vi "Tx handeset.vi"(0 "CMD On":string, 5 "CMD Off":string, 7 "Set Point":string, 9 "Estado do Botão":bool, 11 "Velocity (arcsec/sec)":dbl(slide) min=0.0 scale=0.0..30.0) -> ()   [LabVIEW 2018]
uses:
  Global Tabs.vi
panel:
  out "Offset":dbl min=0.0 max=360.0
  out "mec position":dbl min=0.0 max=360.0 format="%.2f"
  out "pos (deg)":dbl min=0.0 max=360.0 format="%.2f"
  in  "mec pos":dbl min=-22000.0 max=22000.0 step=333.0
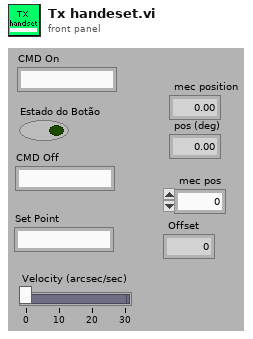
[diagram p1: front panel]
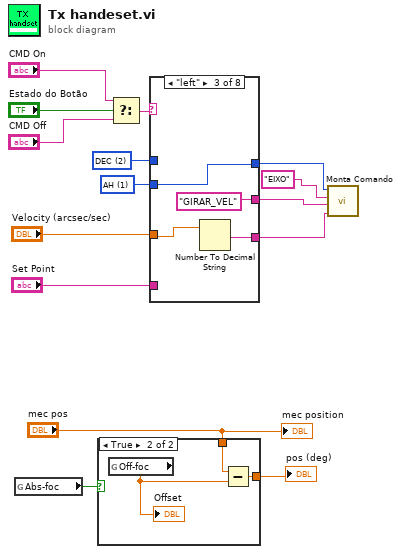
[diagram p0: block diagram]
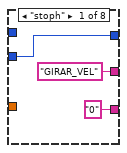
[diagram p3: hidden frame]
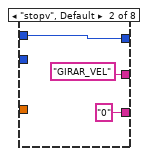
[diagram p4: hidden frame]
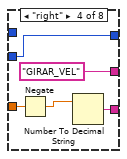
[diagram p5: hidden frame]
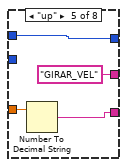
[diagram p6: hidden frame]
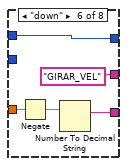
[diagram p7: hidden frame]
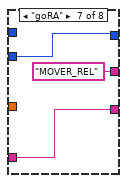
[diagram p8: hidden frame]
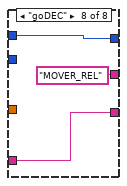
[diagram p9: hidden frame]
diagram:
  w1 = u16 1 items=["ZERO", "AH", "DEC", "TUBO", "CUP"] ("Controlador")
  w2 = u16 2 items=["ZERO", "AH", "DEC", "TUBO", "CUP"] ("Controlador")
  n1 = global read "Global Tabs.vi" "Abs-foc"() -> (w15:bool)
  n2 = case shown="True" w15 {
    tunnel: [w16 w19] -> w13
    tunnel: "mec pos" -> [w16 w18]
    frame False {
    }
    frame True {
      n3 = global read "Global Tabs.vi" "Off-foc"() -> (w17:dbl)
      "Offset" <- w17
      n4 = Subtract(x=w18, y=w17) -> (x-y=w19:dbl)
    }
  }
  "pos (deg)" <- w13
  n5 = Select(t="CMD On", s="Estado do Botão", f="CMD Off") -> (s? t:f=w10:string)
  n6 = case shown="\"left\"" w10 {
    tunnel: [w20 w23 w26 w30 w35 w39 w44 w47] -> w7
    tunnel: "Velocity (arcsec/sec)" -> [_ _ w28 w34 w38 w43 _ _]
    tunnel: ["GIRAR_VEL" ("Comando") "GIRAR_VEL" ("Comando") "GIRAR_VEL" ("Comando") "GIRAR_VEL" ("Comando") "GIRAR_VEL" ("Comando") "GIRAR_VEL" ("Comando") "MOVER_REL" ("Comando") "MOVER_REL" ("Comando")] -> w5
    tunnel: ["0" "0" w29 w32 w37 w42 w46 w49] -> w4
    tunnel: "Set Point" -> [_ _ _ _ _ _ w46 w49]
    tunnel: w2 -> [_ w23 _ _ w35 w39 _ w47]
    tunnel: w1 -> [w20 _ w26 w30 _ _ w44 _]
    frame "stoph" {
    }
    frame "stopv", Default {
    }
    frame "left" {
      n7 = Number To Decimal String(number=w28) -> (decimal integer string=w29:string)  [unwired: 1 in]
    }
    frame "right" {
      n8 = Negate(x=w34) -> (-x=w31:dbl)
      n9 = Number To Decimal String(number=w31) -> (decimal integer string=w32:string)  [unwired: 1 in]
    }
    frame "up" {
      n10 = Number To Decimal String(number=w38) -> (decimal integer string=w37:string)  [unwired: 1 in]
    }
    frame "down" {
      n11 = Negate(x=w43) -> (-x=w41:dbl)
      n12 = Number To Decimal String(number=w41) -> (decimal integer string=w42:string)  [unwired: 1 in]
    }
    frame "goRA" {
    }
    frame "goDEC" {
    }
  }
  n13 = call "Monta Comando.vi"("Set Point"=w4, "Comando"=w5, "Dispositivo"="EIXO" ("Comando"), "Controlador"=w7) -> ()  [unwired: 3 in, 3 out]
  "mec position" <- "mec pos"
